vi "rtin_controlRealTimeInFeedbackLoopMode.vi"(7 "Set":bool, 8 "error in":errorcluster, 9 "mode":i32, 10 "axis in":u8, 11 "connection ID":refnum<k5>) -> (0 "error out":errorcluster, 1 "mode out":i32, 2 "axis out":i32, 3 "connection ID":refnum<k5>)   [LabVIEW 2016]
doc: "Sets or retrieves if the realtime function must operate in closed loop operation or open loop operation"
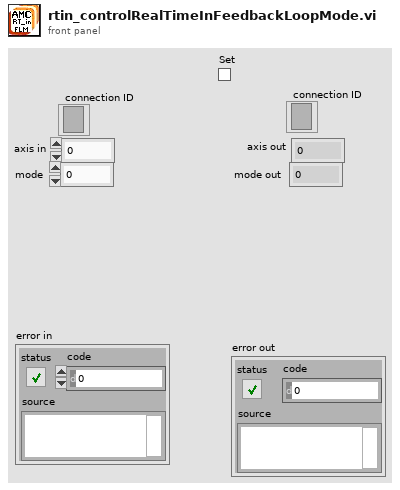
[diagram p1: front panel]
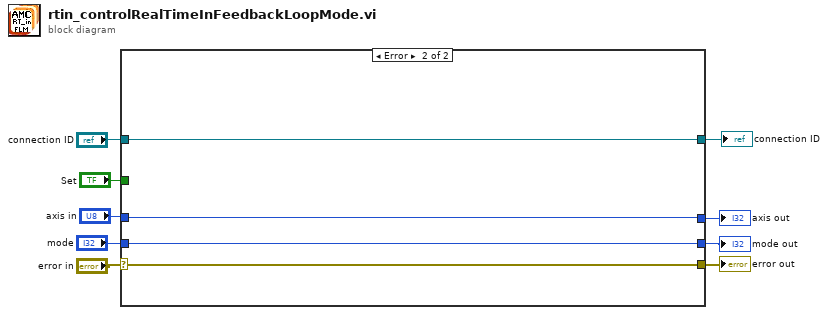
[diagram p0: block diagram]
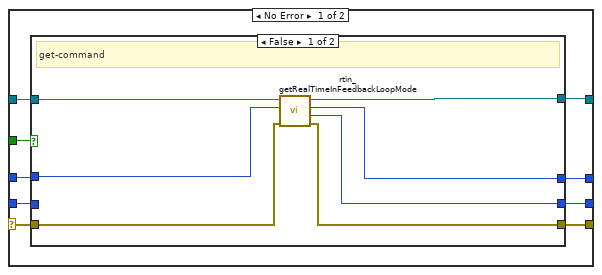
[diagram p2: hidden frame]
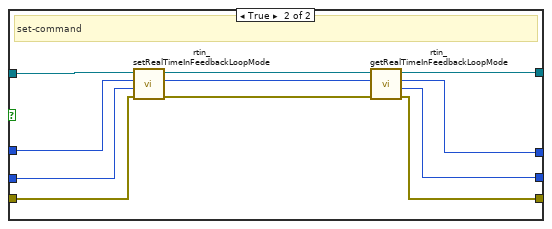
[diagram p3: hidden frame]
diagram:
  n1 = case shown="Error" "error in" {
    selector: "error in" -> [w14 w40]
    tunnel: "axis in" -> [w18 w38]
    tunnel: [w12 w40] -> w8
    tunnel: "mode" -> [w16 w39]
    tunnel: [w13 w39] -> w3
    tunnel: "Set" -> [w15 _]
    tunnel: [w10 w37] -> w6
    tunnel: "connection ID" -> [w17 w37]
    tunnel: [w11 w38] -> w1
    frame No Error {
      n2 = case shown="False" w15 {
        tunnel: w17 -> [w25 w26]
        tunnel: w18 -> [w21 w31]
        tunnel: w16 -> [_ w33]
        tunnel: w14 -> [w22 w36]
        tunnel: [w19 w32] -> w13
        tunnel: [w23 w34] -> w12
        tunnel: [w20 w30] -> w11
        tunnel: [w24 w29] -> w10
        frame False {
          # "get-command"
          n3 = call "rtin_getRealTimeInFeedbackLoopMode.vi"("error in"=w22, "axis"=w21, "connection ID"=w25) -> ("error out"=w23:errorcluster, "mode"=w19:i32, "axis_out"=w20:i32, "connection ID"=w24:refnum<k5>)  [unwired: 5 in]
        }
        frame True {
          # "set-command"
          n4 = call "rtin_setRealTimeInFeedbackLoopMode.vi"("error in"=w36, "mode"=w33, "axis"=w31, "connection ID"=w26) -> ("error out"=w35:errorcluster, "axis_out"=w27:i32, "connection ID"=w28:refnum<k5>)  [unwired: 5 in]
          n5 = call "rtin_getRealTimeInFeedbackLoopMode.vi"("error in"=w35, "axis"=w27, "connection ID"=w28) -> ("error out"=w34:errorcluster, "mode"=w32:i32, "axis_out"=w30:i32, "connection ID"=w29:refnum<k5>)  [unwired: 5 in]
        }
      }
    }
    frame Error {
    }
  }
  "error out" <- w8
  "axis out" <- w1
  "mode out" <- w3
  "connection ID" <- w6
